vi "error.vi"(8 "error in":errorcluster, 11 "channel names":string[](array[string])) -> (0 "error out":errorcluster)   [LabVIEW 2020, in "stream_custom_cluster.lvclass"]
uses:
  stream_custom_cluster.lvclass
  4326555d-cc22-44bd-8e42-8cb6ca847c18.vi
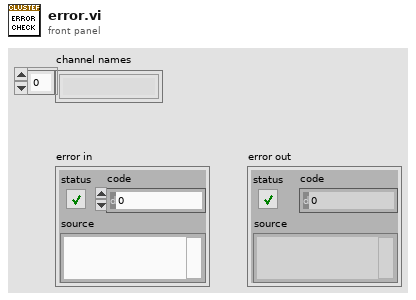
[diagram p1: front panel]
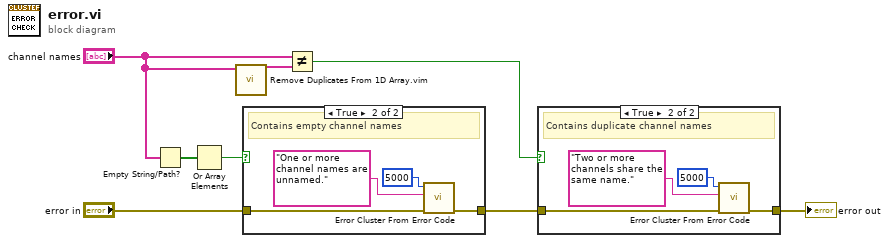
[diagram p0: block diagram]
diagram:
  n1 = Empty String/Path?(string/path="channel names") -> (empty?=w8:bool[])
  n2 = Or Array Elements(Boolean array=w8) -> (logical OR=w7:bool)
  n3 = call "Remove Duplicates From 1D Array.vim"("array"="channel names") -> ("array with duplicates removed"=w5:string[])  [unwired: 10 in]
  n4 = case shown="True" w7 {
    tunnel: "error in" -> [w9 w11]
    tunnel: [w9 w10] -> w2
    frame False {
    }
    frame True {
      # "Contains empty channel names"
      n5 = call <vilib>:"Error Cluster From Error Code.vi"("error in (no error)"=w11, "error message (\"\")"="One or more channel names are unnamed." ("error message (\"\")"), "error code (0)"=5000) -> ("error out"=w10:errorcluster)  [unwired: 6 in]
    }
  }
  n6 = Not Equal?(x="channel names", y=w5) -> (x != y?=w3:bool)
  n7 = case shown="True" w3 {
    tunnel: w2 -> [w14 w16]
    tunnel: [w14 w15] -> w1
    frame False {
    }
    frame True {
      # "Contains duplicate channel names"
      n8 = call <vilib>:"Error Cluster From Error Code.vi"("error in (no error)"=w16, "error message (\"\")"="Two or more channels share the same name." ("error message (\"\")"), "error code (0)"=5000) -> ("error out"=w15:errorcluster)  [unwired: 6 in]
    }
  }
  "error out" <- w1
